vi "T 2 (SubVI).vi"(10 "arg":dbl format="%#_13g") -> (2 "matrix":dbl[][](array[numeric]))   [LabVIEW 2017]
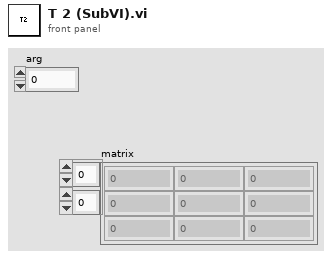
[diagram p1: front panel]
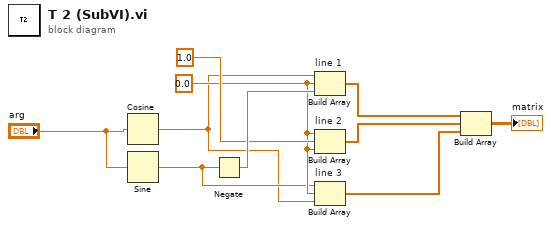
[diagram p0: block diagram]
diagram:
  w3 = 0.0 ("element")
  n1 = Cosine(x="arg") -> (cos(x)=w1:dbl)
  n2 = Sine(x="arg") -> (sin(x)=w2:dbl)
  n3 = Negate(x=w2) -> (-x=w5:dbl)
  n4 = Build Array "line 1"(w1, w3, w5) -> (w7:dbl[])
  n5 = Build Array "line 2"(w3, 1.0 ("element"), w3) -> (w8:dbl[])
  n6 = Build Array "line 3"(w2, w3, w1) -> (w9:dbl[])
  n7 = Build Array(w7, w8, w9) -> (→"matrix":dbl[][])
